vi "Read Step Name.vi"(8 "error in (no error)":errorcluster, 11 "StepNode in":refnum<class "StepNode.lvclass">) -> (0 "error out":errorcluster, 2 "Step Name":string, 3 "StepNode out":refnum<class "StepNode.lvclass">)   [LabVIEW 2015, in "StepNode.lvclass"]
uses:
  StepNode.lvclass
  StepNode.lvclass/StepNode.ctl
  Prototype/classes/Step/Config/Step Config.lvclass
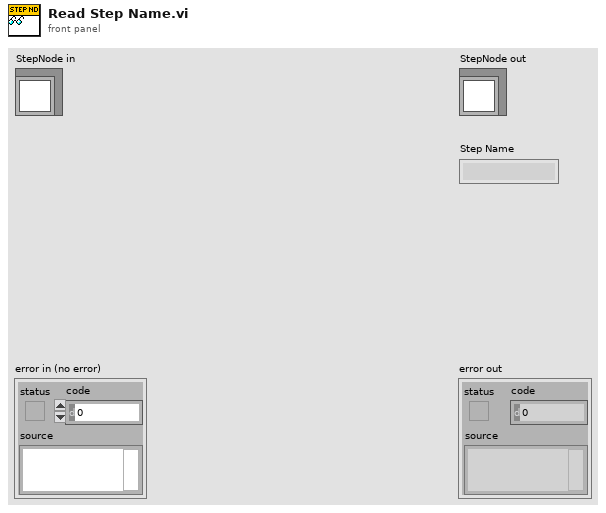
[diagram p1: front panel]
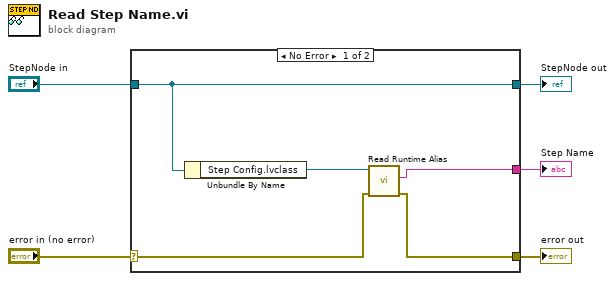
[diagram p0: block diagram]
diagram:
  n1 = case shown="No Error" "error in (no error)" {
    selector: "error in (no error)" -> [w7 w11]
    tunnel: [w6 w11] -> w4
    tunnel: [w10 w12] -> w2
    tunnel: "StepNode in" -> [w10 w12]
    tunnel: [w8 _] -> w1
    frame No Error {
      n2 = Unbundle By Name(w10) -> ("Step Config.lvclass"=w9:refnum<class "Step Config.lvclass">)
      n3 = call-dynamic "Read Runtime Alias.vi"("error in (no error)"=w7, "Step Config in"=w9) -> ("error out"=w6:errorcluster, "Runtime Alias"=w8:string)  [unwired: 7 in, 1 out]
    }
    frame Error {
    }
  }
  "error out" <- w4
  "StepNode out" <- w2
  "Step Name" <- w1
